vi "parseDataDBLArray.vi"(0 "U8ArrayParserAutoIndexing in":refnum<class "U8ArrayParserAutoIndexing.lvclass">, 1 "Length":i32, 2 "OverrideSwapBytes":bool, 3 "error in (no error)":errorcluster) -> (7 "U8ArrayParserAutoIndexing out":refnum<class "U8ArrayParserAutoIndexing.lvclass">, 8 "Data":dbl[](array[numeric]), 10 "error out":errorcluster)   [LabVIEW 2016, in "RTUtilities.lvlib" / "U8ArrayParserAutoIndexing.lvclass"]
uses:
  U8ArrayParserAutoIndexing.lvclass
  U8ArrayParserAutoIndexing.lvclass/U8ArrayParserAutoIndexing.ctl
  U8ArrayParser/U8ArrayParserManualIndexing.lvclass
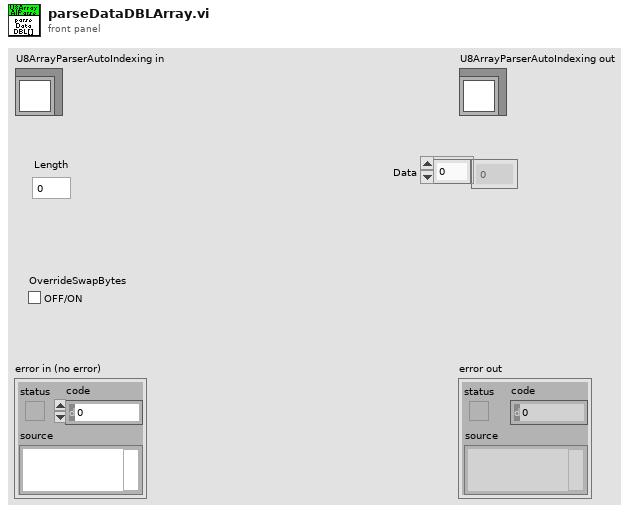
[diagram p1: front panel]
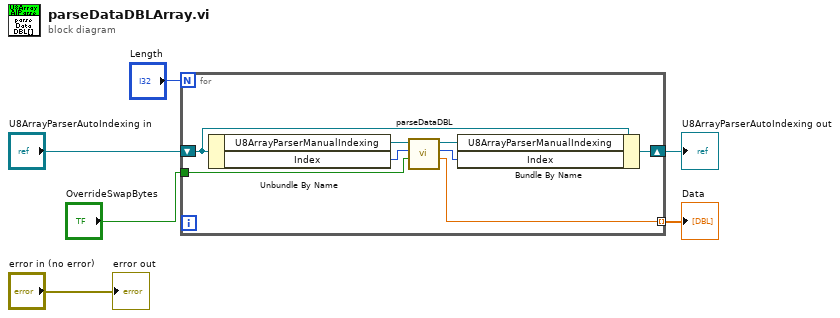
[diagram p0: block diagram]
diagram:
  n1 = for {
    N: "Length" -> [_]
    shift-right: [w9] -> w4
    shift-left: "U8ArrayParserAutoIndexing in" -> [w12]
    tunnel: "OverrideSwapBytes" -> [w8]
    tunnel: [w7] -> w1 mode=indexing
    n2 = Unbundle By Name(w12) -> ("U8ArrayParserManualIndexing"=w14:refnum<class "U8ArrayParserManualIndexing.lvclass">, "Index"=w13:i32)
    n3 = call "parseDataDBL.vi"("OverrideSwapBytes"=w8, "Index"=w13, "U8ArrayParserManualIndexing in"=w14) -> ("Data"=w7:dbl, "Index out"=w10:i32, "U8ArrayParserManualIndexing out"=w11:refnum<class "U8ArrayParserManualIndexing.lvclass">)  [unwired: 5 in, 1 out]
    n4 = Bundle By Name(cluster=w12, "U8ArrayParserManualIndexing"=w11, "Index"=w10) -> (w9:refnum<class "U8ArrayParserAutoIndexing.lvclass">)
  }
  "U8ArrayParserAutoIndexing out" <- w4
  "Data" <- w1
  "error out" <- "error in (no error)"
